vi "Do.vi"(8 "error in (no error)":errorcluster, 10 "Actor in":refnum<class "Actor.lvclass">, 11 "Change Oven Type Msg":refnum<class "Change Oven Type Msg.lvclass">) -> (0 "error out":errorcluster, 2 "Actor out":refnum<class "Actor.lvclass">)   [LabVIEW 2021, in "Oven Actor.lvlib" / "Change Oven Type Msg.lvclass"]
doc: "This VI delivers the message to the actor by calling the appropriate method(s) on the actor."
uses:
  Change Oven Type Msg.lvclass
  e64065c6-bf5a-4917-b7cf-b0b00c28c54c.vi
  Oven Actor/Oven Actor.lvclass
  <vilib>/ActorFramework/Actor/Actor.lvclass
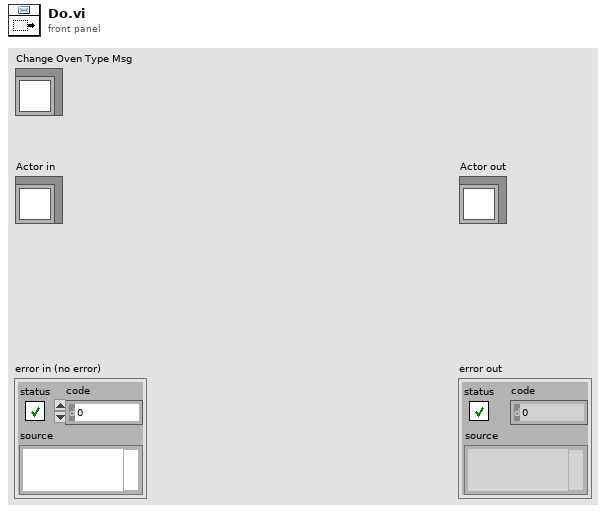
[diagram p1: front panel]
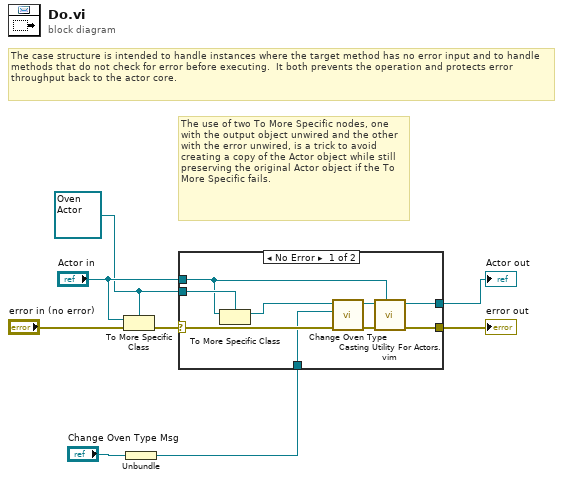
[diagram p0: block diagram]
diagram:
  w3 = refnum<class "Oven Actor.lvclass"> refnum ("Actor in")
  # "The use of two To More Specific nodes, one with the output object unwired and the other with the error unwired, is a trick to avoid creating a copy of the Actor object while still preserving the original Actor object if the To More Specific fails."
  # "The case structure is intended to handle instances where the target method has no error input and to handle methods that do not check for error before executing.  It both prevents the operation and protects error throughput back to the actor core."
  n1 = To More Specific Class(target class=w3, reference="Actor in", error in="error in (no error)") -> (error out=w2:errorcluster)  [unwired: 1 out]
  n2 = Unbundle("Change Oven Type Msg") -> (w1:refnum<class "Oven Actor.lvclass">)
  n3 = case shown="No Error" w2 {
    selector: w2 -> [w17 w19]
    tunnel: [w12 w19] -> w8
    tunnel: [w13 w18] -> w7
    tunnel: "Actor in" -> [w15 w18]
    tunnel: w3 -> [w16 _]
    tunnel: w1 -> [w9 _]
    frame No Error {
      n4 = To More Specific Class(target class=w16, reference=w15) -> (specific class reference=w10:refnum<class "Oven Actor.lvclass">)  [unwired: 1 in, 1 out]
      n5 = call "Change Oven Type.vi"("error in (no error)"=w17, "New Oven Type"=w9, "Oven Actor in"=w10) -> ("error out"=w11:errorcluster, "Oven Actor out"=w14:refnum<class "Oven Actor.lvclass">)  [unwired: 7 in]
      n6 = call "Casting Utility For Actors.vim"("type"=w15, "error in (no error)"=w11, "Actor in"=w14) -> ("error out"=w12:errorcluster, "Actor out"=w13:refnum<class "Actor.lvclass">)  [unwired: 7 in]
    }
    frame Error {
      # "If type check fails, pass the original object out again."
    }
  }
  "error out" <- w8
  "Actor out" <- w7
